vi "GetObjectCount.vi"(8 "error in (no error)":errorcluster, 11 "Scene Object In":refnum<vi>) -> (0 "error out":errorcluster, 2 "all objects":refnum<vi>[](array[refnum]), 3 "object count":i32)   [LabVIEW 2014]
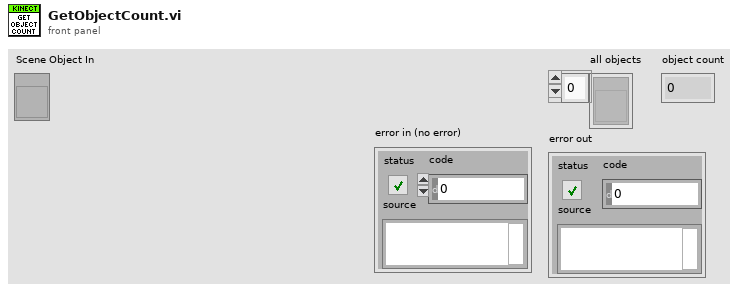
[diagram p1: front panel]
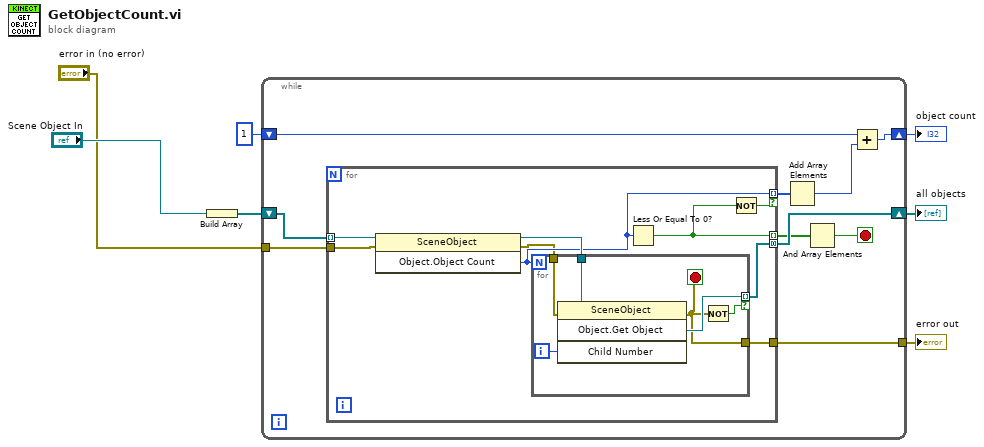
[diagram p0: block diagram]
diagram:
  n1 = Build Array("Scene Object In") -> (w7:refnum<vi>[])
  n2 = while {
    shift-right: [w16] -> w4
    shift-left: w7 -> [w17]
    shift-right: [w11] -> w3
    shift-left: 1 -> [w10]
    tunnel: [w9] -> w2
    tunnel: "error in (no error)" -> [w8]
    stop <- w14 stop-if-true
    n3 = for {
      tunnel: w17 -> [w26] mode=indexing
      tunnel: [w24] -> w16 mode=concatenating
      tunnel: [w21] -> w15 mode=indexing
      tunnel: [w23] -> w13 mode=indexing if=w22
      tunnel: [w19] -> w9
      tunnel: w8 -> [w18]
      n4 = invoke class="SceneObject" method="Object.Object Count"(reference=w26, error in=w18) -> (reference out=w25:refnum<vi>, error out=w20:errorcluster, "Child Count"=w23:i32)  [unwired: 1 in]
      n5 = for {
        N: w23 -> [_]
        tunnel: w25 -> [w32]
        tunnel: [w30] -> w24 mode=indexing if=w29
        tunnel: w20 -> [w28]
        tunnel: [w27] -> w19
        i -> [w31]
        stop <- w27 stop-if-true
        n6 = invoke class="SceneObject" method="Object.Get Object"(reference=w32, error in=w28, "Child Number"=w31) -> (error out=w27:errorcluster, "Get Child"=w30:refnum<vi>)  [unwired: 1 in, 2 out]
        n7 = Not(x=w27) -> (.not. x?=w29:bool)
      }
      n8 = Less Or Equal To 0?(x=w23) -> (x <= 0?=w21:bool)
      n9 = Not(x=w21) -> (.not. x?=w22:bool)
    }
    n10 = Add Array Elements(numeric array=w13) -> (sum=w12:i32)
    n11 = And Array Elements(Boolean array=w15) -> (logical AND=w14:bool)
    n12 = Add(x=w10, y=w12) -> (x+y=w11:i32)
  }
  "all objects" <- w4
  "object count" <- w3
  "error out" <- w2
